vi "Undistort.vi"   [LabVIEW 2020, in "image.lvlib"]
uses:
  image.lvlib
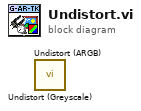
[diagram p0: block diagram]
diagram:
  n1 = call "Undistort (Greyscale).vi"() -> ()  [unwired: 10 in, 2 out]
  n2 = call "Undistort (ARGB).vi"() -> ()  [unwired: 10 in, 2 out]
